vi "User_Console.vi"(8 "error in (no error)":errorcluster) -> (0 "error out":errorcluster)   [LabVIEW 2020]
doc: "Thread VIT"
uses:
  controls/Event_User.ctl
  controls/Configuration_Database.ctl
  controls/Share_Data.ctl
  <vilib>/Utility/error.llb/Error Cluster From Error Code.vi
  <vilib>/ErrorRing/Error Ring.xnode
  SubVIs/Message Queue/Message Queue.lvlib
  controls/FGV_To_Do.ctl
  Controller/User_Console_Local_Data.ctl
  Controller/User_Console_References.ctl
  SubVIs/Message Queue/Enqueue Message (Single).vi
  Controller/User_Console.ctl
panel:
  in  "User Console":T1
  # "[Covers: UI1]"
  # "[Covers: UI12A]"
  # "[Covers: UI12A1]"
  # "[Covers: UI12B]"
  # "[Covers: UI12B1]"
  # "[Covers: UI12A2]"
  # "[Covers: UI12B2]"
  # "[Covers: UI2D]"
  # "[Covers: UI2D1]"
  # "Fourth Floor"
  # "Third Floor"
  # "Second Floor"
  # "First Floor"
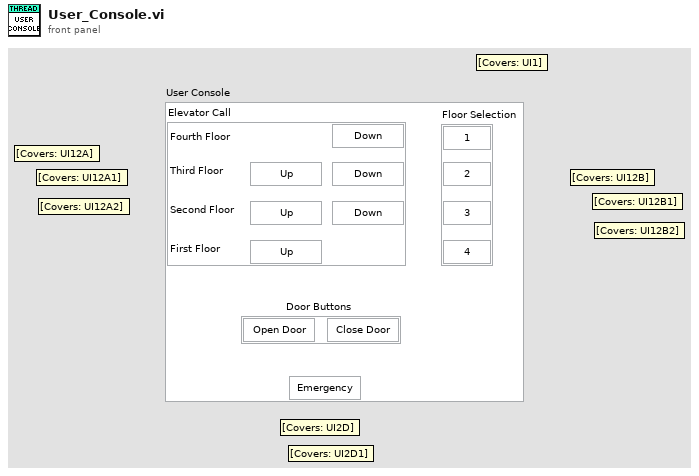
[diagram p1: front panel]
types:
  T1 = typedef "User_Console.ctl" = cluster{"Elevator Call":cluster{"Fourth Floor Down":bool, "Third Floor Down":bool, "Second Floor Down":bool, "Third Floor Up":bool, "Second Floor Up":bool, "First Floor Up":bool}, "Floor Selection":cluster{"1":bool, "2":bool, "3":bool, "4":bool}, "Door Buttons":cluster{"OpenDoor":bool, "CloseDoor":bool}, "Emergency":bool}
  T2 = typedef "FGV_To_Do.ctl" = enum16{"1 - Initialize_Events", "2 - Read_Database", "3 - Initialize QMH", "Save_Database", "Read", "4 - Close_Events", "5 - Close_QMH"}
  T3 = typedef "All_Communication_Data.ctl" = cluster{"ConfigurationDatabase":T4, "QMH":T5, "User Event":T6}
  T4 = typedef "Configuration_Database.ctl" = cluster{"DoorOpen":u8, "DoorClose":u8, "TravelTime":u8, "InactivityTime":u8}
  T5 = typedef "Message Queue.lvlib/All Message Queues.ctl" = cluster{"UserConsole":refnum<queue>, "DisplayConsole":refnum<queue>, "SensorInterface":refnum<queue>}
  T6 = typedef "Event_User.ctl" = cluster{"User Event - Stop":refnum<user-event>, "User Event - Error":refnum<user-event>}
  T7 = typedef "User_Console_Local_Data.ctl" = cluster{"Configuration_Data":T8, "UserConsole_Ref":T9, "Travel?":bool, "Terminate?":bool, "Inactivity time":dbl}
  T8 = typedef "Share_Data.ctl" = cluster{"ConfigurationDatabase":T4, "User Event":T6}
  T9 = typedef "User_Console_References.ctl" = cluster{"First Floor Up":refnum<vi>, "Second Floor Up":refnum<vi>, "Third Floor Up":refnum<vi>, "Second Floor Down":refnum<vi>, "Third Floor Down":refnum<vi>, "Fourth Floor Down":refnum<vi>, "1":refnum<vi>, "2":refnum<vi>, "3":refnum<vi>, "4":refnum<vi>, "Emergency":refnum<vi>, "CloseDoor":refnum<vi>, "OpenDoor":refnum<vi>}
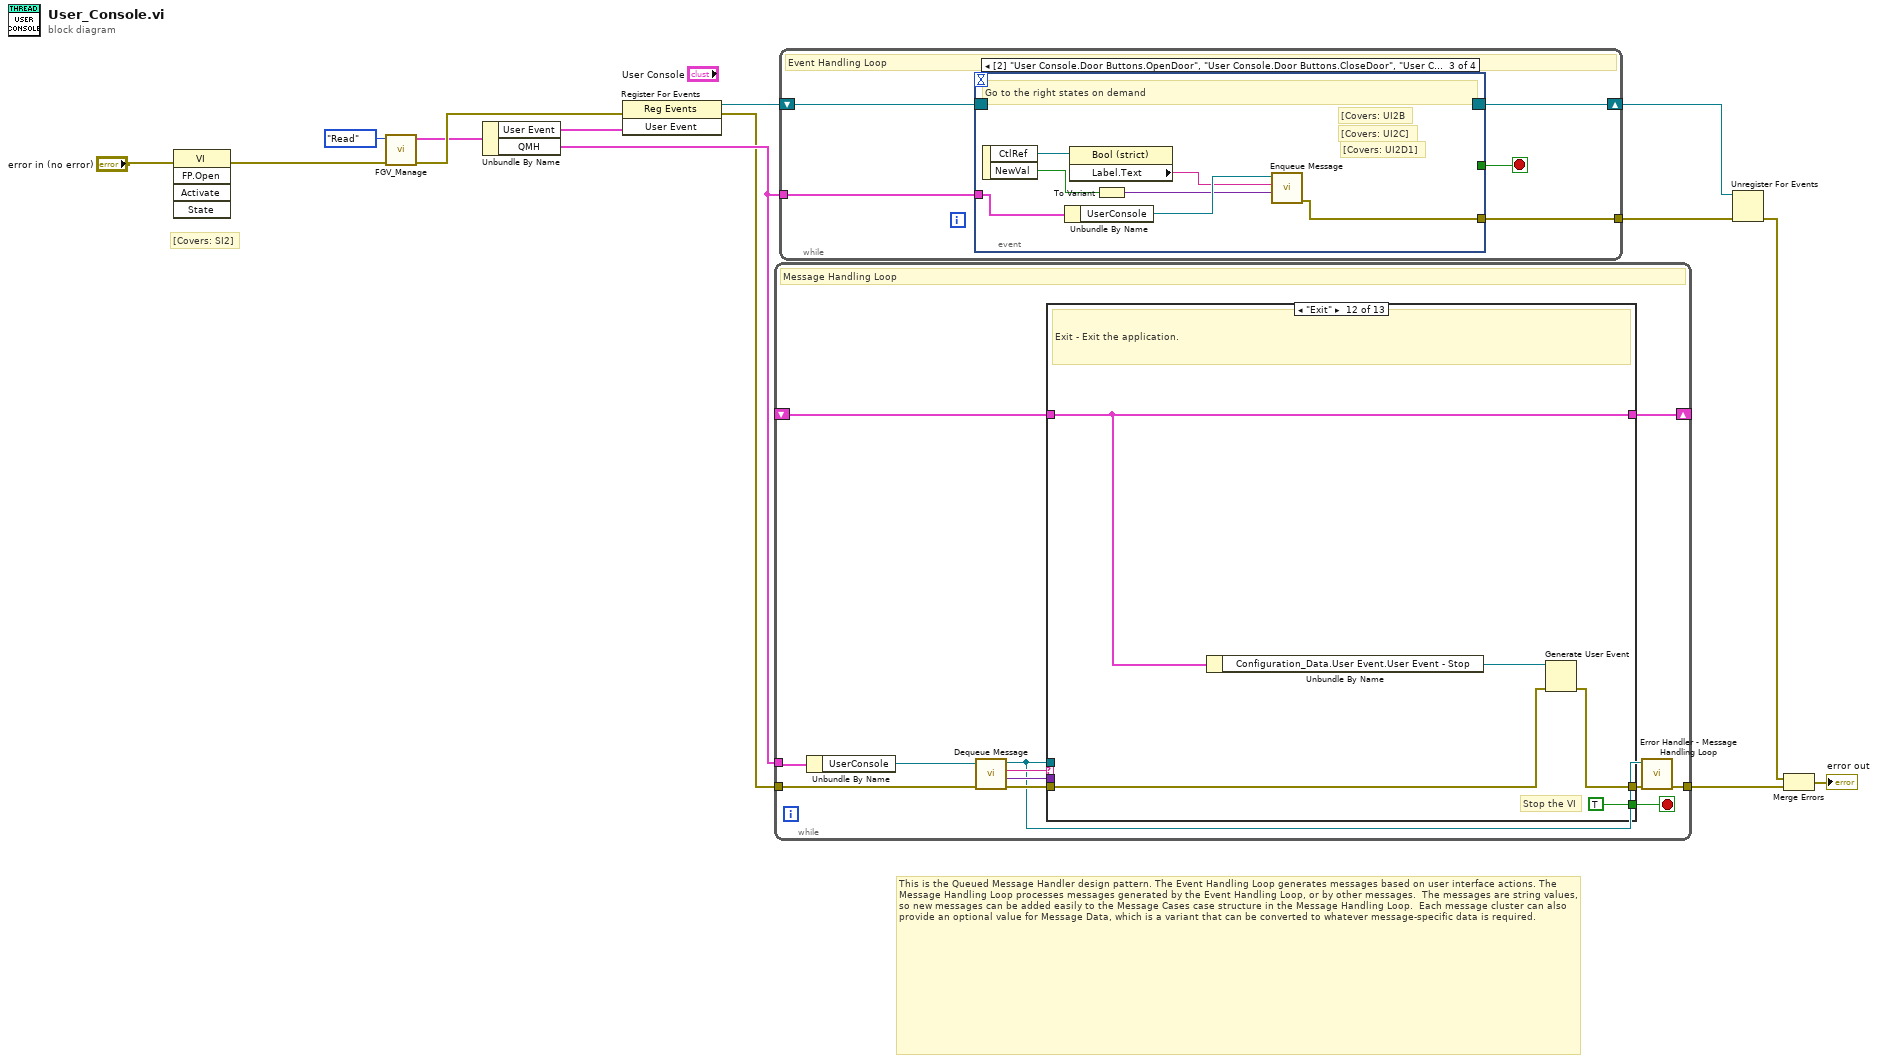
[diagram p0: block diagram]
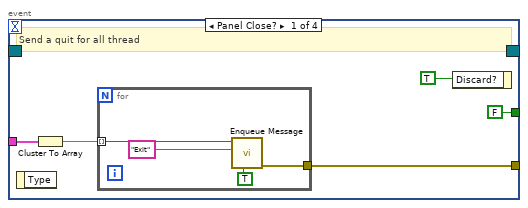
[diagram p2: hidden frame]
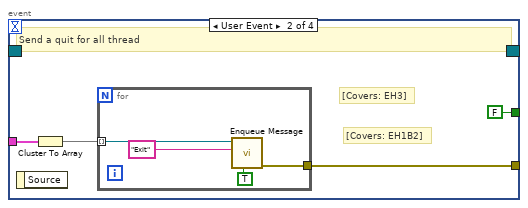
[diagram p3: hidden frame]
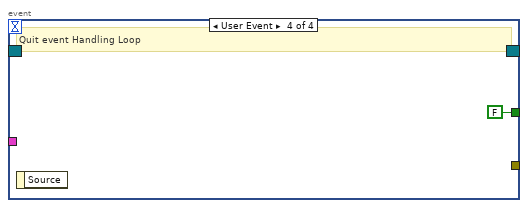
[diagram p4: hidden frame]
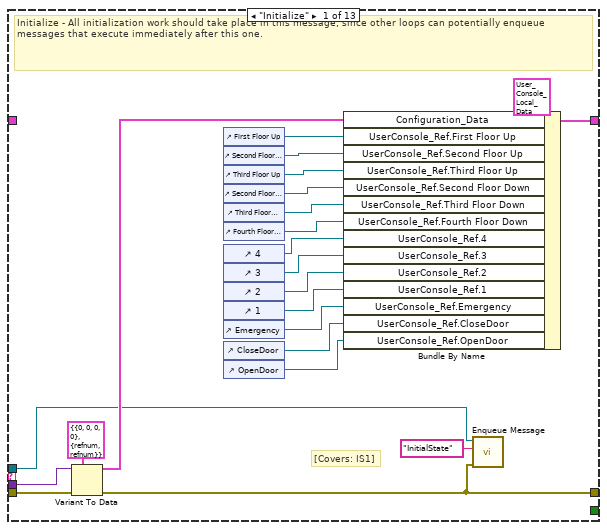
[diagram p5: hidden frame]
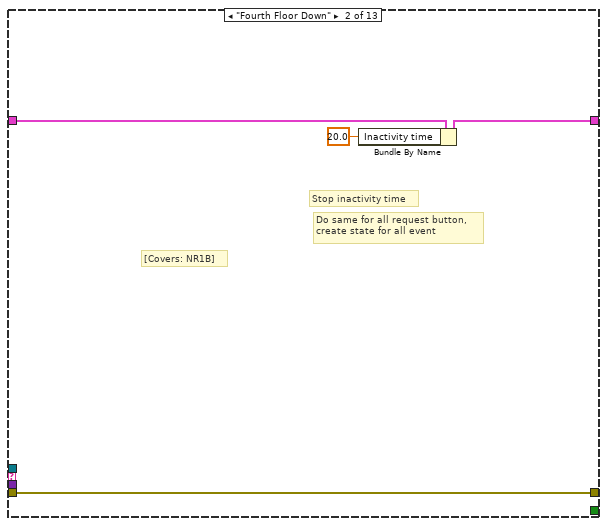
[diagram p6: hidden frame]
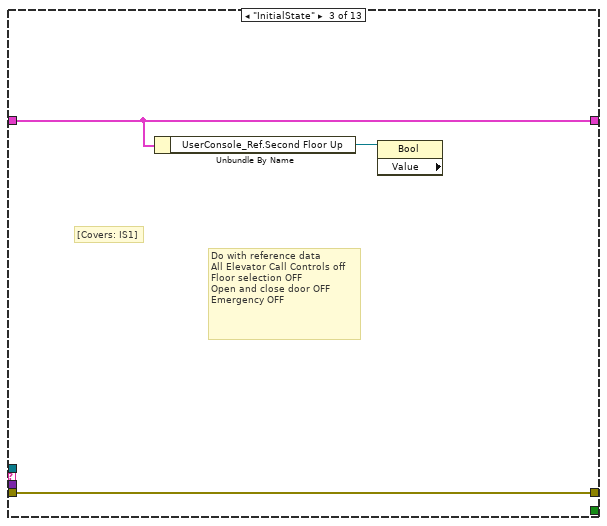
[diagram p7: hidden frame]
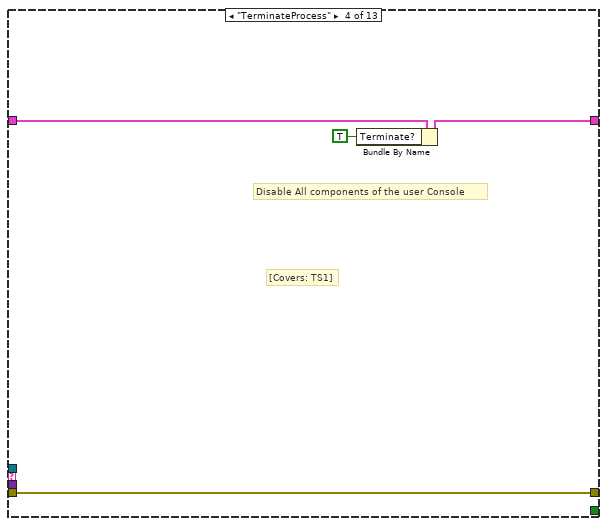
[diagram p8: hidden frame]
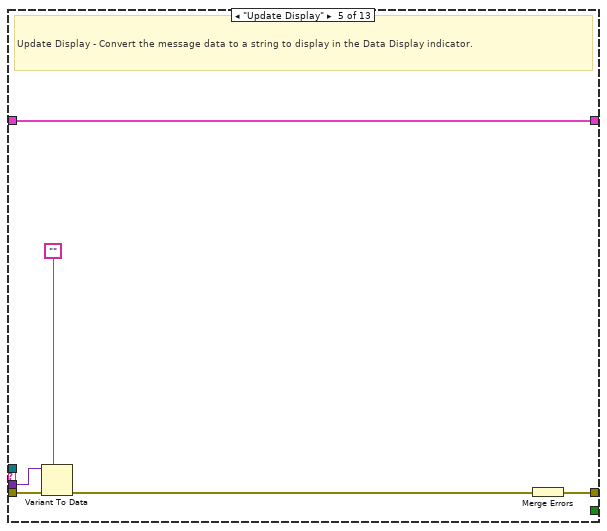
[diagram p9: hidden frame]
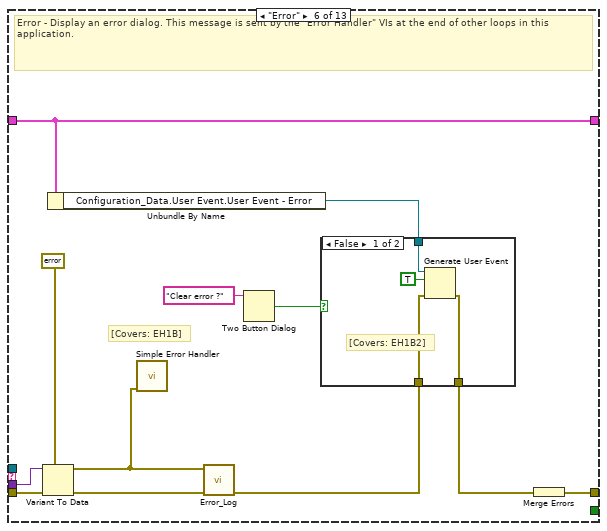
[diagram p10: hidden frame]
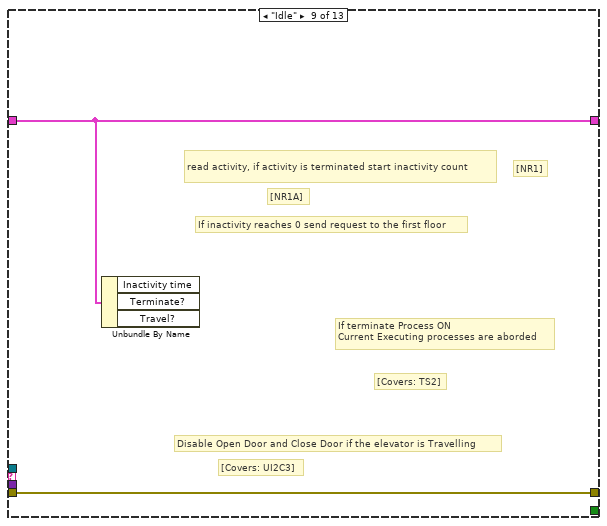
[diagram p14: hidden frame]
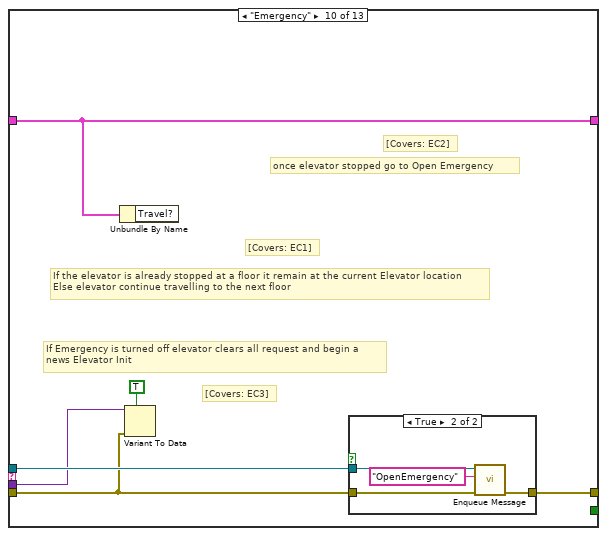
[diagram p15: hidden frame]
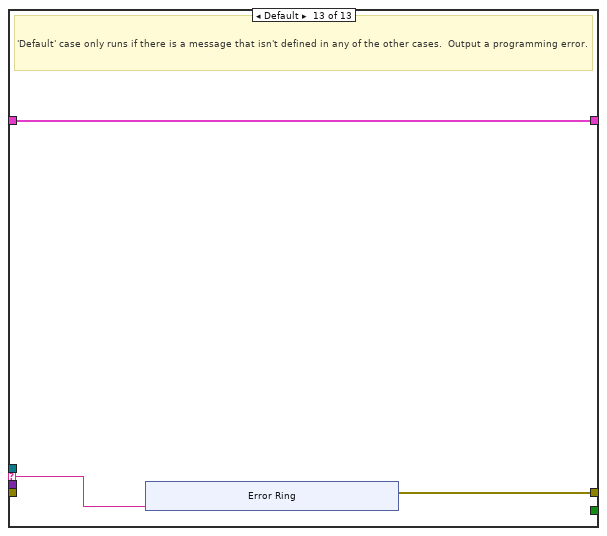
[diagram p18: hidden frame]
diagram:
  # "[Covers: SI2]"
  # "This is the Queued Message Handler design pattern. The Event Handling Loop generates messages based on user interface actions. The Message Handling Loop processes messages generated by the Event Handling Loop, or by other messages.  The messages are string values, so new messages can be added easily to the Message Cases case structure in the Message Handling Loop.  Each message cluster can also provide an optional value for Message Data, which is a variant that can be converted to whatever message-specific data is required."
  n1 = invoke class="VI" method="FP.Open"(error in="error in (no error)") -> (error out=w1:errorcluster)  [unwired: 4 in, 4 out]
  n2 = call "FGV_Manage.vi"("error in (no error)"=w1, "To do"=FGV_To_Do."Read") -> ("error out"=w11:errorcluster, "All_Communication OUT"=w9:T3)  [unwired: 8 in]
  n3 = Unbundle By Name(w9) -> ("User Event"=w10:T6, "QMH"=w13:T5)
  n4 = register-events(error in=w11, w10) -> (reference out=w7:refnum<event-registration>, error out=w12:errorcluster)  [unwired: 1 in]
  n5 = while {
    tunnel: w13 -> [w16]
    shift-right: [w25] -> _
    shift-left: _ -> [w26]
    tunnel: w12 -> [w23]
    tunnel: [w18] -> w3
    stop <- w24 stop-if-true
    # "Message Handling Loop"
    n6 = Unbundle By Name(w16) -> ("UserConsole"=w15:refnum<queue>)
    n7 = call "Dequeue Message.vi"("error in (no error)"=w23, "Message Queue"=w15) -> ("error out"=w22:errorcluster, "Message Data"=w20:variant, "Message"=w21:string, "dup Message Queue"=w19:refnum<queue>)  [unwired: 6 in]
    n8 = case "Message Cases" shown="\"Exit\"" w21 {
      selector: w21 -> [_ _ _ _ _ _ _ _ _ _ _ _ w106]
      tunnel: w19 -> [w28 _ _ _ _ _ _ _ _ w92 _ _ _]
      tunnel: w22 -> [w47 w52 w55 w59 w63 w77 w84 w86 w88 w91 w100 w102 _]
      tunnel: [w29 w52 w55 w59 w64 w74 w84 w86 w88 w93 w100 w101 w107] -> w17
      tunnel: w26 -> [_ w51 w54 w58 w65 w71 w83 w85 w87 w94 w99 w104 w108]
      tunnel: [w43 w50 w54 w57 w65 w71 w83 w85 w87 w94 w99 w104 w108] -> w25
      tunnel: [_ _ _ _ _ _ _ _ _ _ _ TRUE _] -> w24
      tunnel: w20 -> [w46 _ _ _ w62 w76 _ _ _ w90 _ _ _]
      frame "Initialize" {
        # "[Covers: IS1]"
        # "Initialize - All initialization work should take place in this message, since other loops can potentially enqueue messages that execute immediately after this one."
        n9 = Variant To Data(error in=w47, type=T8 {"ConfigurationDatabase"={"DoorOpen"=0, "DoorClose"=0, "TravelTime"=0, "InactivityTime"=0}, "User Event"={"User Event - Stop"=refnum, "User Event - Error"=refnum}} ("Share_Data"), Variant=w46) -> (data=w44:T8, error out=w29:errorcluster)
        n10 = control-ref of="First Floor Up"() -> (w42:refnum<vi>)
        n11 = control-ref of="Second Floor Up"() -> (w41:refnum<vi>)
        n12 = control-ref of="Third Floor Up"() -> (w40:refnum<vi>)
        n13 = control-ref of="Second Floor Down"() -> (w39:refnum<vi>)
        n14 = control-ref of="Third Floor Down"() -> (w38:refnum<vi>)
        n15 = control-ref of="Fourth Floor Down"() -> (w37:refnum<vi>)
        n16 = control-ref of="4"() -> (w36:refnum<vi>)
        n17 = control-ref of="3"() -> (w35:refnum<vi>)
        n18 = control-ref of="2"() -> (w34:refnum<vi>)
        n19 = control-ref of="1"() -> (w33:refnum<vi>)
        n20 = control-ref of="Emergency"() -> (w32:refnum<vi>)
        n21 = control-ref of="CloseDoor"() -> (w31:refnum<vi>)
        n22 = control-ref of="OpenDoor"() -> (w30:refnum<vi>)
        n23 = Bundle By Name(cluster=T7 {"Configuration_Data"={"ConfigurationDatabase"={"DoorOpen"=0, "DoorClose"=0, "TravelTime"=0, "InactivityTime"=0}, "User Event"={"User Event - Stop"=refnum, "User Event - Error"=refnum}}, "UserConsole_Ref"={"First Floor Up"=refnum, "Second Floor Up"=refnum, "Third Floor Up"=refnum, "Second Floor Down"=refnum, "Third Floor Down"=refnum, "Fourth Floor Down"=refnum, "1"=refnum, "2"=refnum, "3"=refnum, "4"=refnum, "Emergency"=refnum, "CloseDoor"=refnum, "OpenDoor"=refnum}, "Travel?"=FALSE, "Terminate?"=FALSE, "Inactivity time"=0.0} ("Local_Data"), "Configuration_Data"=w44, "UserConsole_Ref.First Floor Up"=w42, "UserConsole_Ref.Second Floor Up"=w41, "UserConsole_Ref.Third Floor Up"=w40, "UserConsole_Ref.Second Floor Down"=w39, "UserConsole_Ref.Third Floor Down"=w38, "UserConsole_Ref.Fourth Floor Down"=w37, "UserConsole_Ref.4"=w36, "UserConsole_Ref.3"=w35, "UserConsole_Ref.2"=w34, "UserConsole_Ref.1"=w33, "UserConsole_Ref.Emergency"=w32, "UserConsole_Ref.CloseDoor"=w31, "UserConsole_Ref.OpenDoor"=w30) -> (w43:T7)
        n24 = call-poly "Enqueue Message.vi"("error in (no error)"=w29, "Message"="InitialState", "Message Queue"=w28) -> ()  [unwired: 7 in, 2 out]
      }
      frame "Fourth Floor Down" {
        # "Do same for all request button, \ncreate state for all event"
        # "Stop inactivity time"
        # "[Covers: NR1B]"
        n25 = Bundle By Name(cluster=w51, "Inactivity time"=20.0) -> (w50:T7)
      }
      frame "InitialState" {
        # "[Covers: IS1]"
        # "Do with reference data\nAll Elevator Call Controls off\nFloor selection OFF\nOpen and close door OFF\nEmergency OFF"
        n26 = Unbundle By Name(w54) -> ("UserConsole_Ref.Second Floor Up"=w53:refnum<vi>)
        n27 = property class="Bool" props=["Value"](reference=w53) -> ()  [unwired: 1 in, 3 out]
      }
      frame "TerminateProcess" {
        # "[Covers: TS1]"
        # "Disable All components of the user Console"
        n28 = Bundle By Name(cluster=w58, "Terminate?"=TRUE) -> (w57:T7)
      }
      frame "Update Display" {
        # "Update Display - Convert the message data to a string to display in the Data Display indicator."
        n29 = Variant To Data(error in=w63, type="", Variant=w62) -> (error out=w60:errorcluster)  [unwired: 1 out]
        n30 = Merge Errors(w60) -> (w64:errorcluster)
      }
      frame "Error" {
        # "[Covers: EH1B]"
        # "Error - Display an error dialog. This message is sent by the \"Error Handler\" VIs at the end of other loops in this application."
        n31 = Variant To Data(error in=w77, type=errorcluster {"status"=FALSE, "code"=0, "source"=""} ("error constant"), Variant=w76) -> (data=w72:errorcluster, error out=w73:errorcluster)
        n32 = Unbundle By Name(w71) -> ("Configuration_Data.User Event.User Event - Error"=w70:refnum<user-event>)
        n33 = call <vilib>:"Simple Error Handler.vi"("error in (no error)"=w72) -> ()  [unwired: 4 in, 5 out]
        n34 = call "Error_Log.vi"("error in"=w73, "Error report"=w72) -> ("error out"=w67:errorcluster)  [unwired: 9 in]
        n35 = Two Button Dialog(message="Clear error ?") -> (T button?=w69:bool)  [unwired: 2 in]
        n36 = case shown="False" w69 {
          tunnel: w70 -> [w81 _]
          tunnel: w67 -> [w79 w82]
          tunnel: [w78 w82] -> w66
          frame False {
            # "[Covers: EH1B2]"
            n37 = Generate User Event(user event=w81, event data cluster=TRUE ("event data"), error in=w79) -> (error out=w78:errorcluster)  [unwired: 1 in, 1 out]
          }
          frame True {
            # "[Covers: EH1B1]"
          }
        }
        n38 = Merge Errors(w66) -> (w74:errorcluster)
      }
      frame "OpenDoor" {
        # "[Covers: UI2C1]"
        # "Open Door when the elevator is stopped on a floor"
      }
      frame "CloseDoor" {
        # "[Covers: UI2C2]"
        # "Close Door when the elevator is stopped on a floor"
      }
      frame "Idle" {
        # "read activity, if activity is terminated start inactivity count"
        # "[NR1A]"
        # "If inactivity reaches 0 send request to the first floor"
        # "[NR1]"
        # "[Covers: TS2]"
        # "If terminate Process ON\nCurrent Executing processes are aborded"
        # "Disable Open Door and Close Door if the elevator is Travelling"
        # "[Covers: UI2C3]"
        n39 = Unbundle By Name(w87) -> ()  [unwired: 3 out]
      }
      frame "Emergency" {
        # "[Covers: EC3]"
        # "If Emergency is turned off elevator clears all request and begin a \nnews Elevator Init"
        # "once elevator stopped go to Open Emergency"
        # "[Covers: EC2]"
        # "If the elevator is already stopped at a floor it remain at the current Elevator location\nElse elevator continue travelling to the next floor"
        # "[Covers: EC1]"
        n40 = Unbundle By Name(w94) -> ()  [unwired: 1 out]
        n41 = Variant To Data(error in=w91, type=TRUE, Variant=w90) -> ()  [unwired: 2 out]
        n42 = case shown="True" {
          selector: _ -> [_ _]
          tunnel: [_ w98] -> w93
          tunnel: w92 -> [_ w97]
          tunnel: w91 -> [_ w95]
          frame False {
          }
          frame True {
            n43 = call-poly "Enqueue Message.vi"("error in (no error)"=w95, "Message"="OpenEmergency", "Message Queue"=w97) -> ("error out"=w98:errorcluster)  [unwired: 7 in, 1 out]
          }
        }
      }
      frame "OpenEmergency" {
        # "Door Open and remain Open"
        # "[Covers: EC2]"
      }
      frame "Exit" {
        # "Stop the VI"
        # "Exit - Exit the application."
        n44 = Unbundle By Name(w104) -> ("Configuration_Data.User Event.User Event - Stop"=w103:refnum<user-event>)
        n45 = Generate User Event(user event=w103, error in=w102) -> (error out=w101:errorcluster)  [unwired: 2 in, 1 out]
      }
      frame Default {
        # "'Default' case only runs if there is a message that isn't defined in any of the other cases.  Output a programming error."
        n46 = xnode "Error Ring"("parameter 0"=w106) -> ("error out"=w107:errorcluster)
      }
    }
    n47 = call "Error Handler - Message Handling Loop.vi"("error in (no error)"=w17, "Message Queue"=w19) -> ("dup error in"=w18:errorcluster)  [unwired: 8 in, 1 out]
  }
  n48 = while {
    tunnel: w13 -> [w120]
    shift-right: [w118] -> w5
    shift-left: w7 -> [w119]
    tunnel: [w116] -> w6
    stop <- w117 stop-if-true
    # "Event Handling Loop"
    n49 = event shown="[2] \"User Console.Door Buttons.OpenDoor\", \"User Console.Door Buttons.CloseDoor\", \"User Console.Emergency\", \"User Console.Floor Selection.1\", \"User Console.Floor Selection.2\", \"User Console.Floor Selection.3\", \"User Console.Floor Selection.4\": Value Change" {
      selector: w119 -> [_ _ _ _]
      dyn-events: [_ _ _ _] -> w118
      timeout: _ -> [_ _ _ _]
      tunnel: [FALSE ("Discard?") FALSE ("Discard?") _ FALSE ("Discard?")] -> w117
      tunnel: w120 -> [w124 w133 w143 _]
      tunnel: [w123 w132 w140 _] -> w116
      event Panel Close? {
        # "Send a quit for all thread"
        n50 = event-data() -> ()  [unwired: 1 in, 1 out]
        n51 = Cluster To Array(cluster=w124) -> (array=w122:refnum<queue>[])
        n52 = for {
          tunnel: w122 -> [w129] mode=indexing
          tunnel: [w128] -> w123
          n53 = call-poly "Enqueue Message.vi"("Priority Message? (F)"=TRUE, "Message"="Exit", "Message Queue"=w129) -> ("error out"=w128:errorcluster)  [unwired: 7 in, 1 out]
        }
        n54 = event-data("Discard?"=TRUE) -> ()  [unwired: 1 in, 1 out]
      }
      event User Event {
        # "[Covers: EH3]"
        # "[Covers: EH1B2]"
        # "Send a quit for all thread"
        n55 = event-data() -> ()  [unwired: 1 in, 1 out]
        n56 = Cluster To Array(cluster=w133) -> (array=w131:refnum<queue>[])
        n57 = for {
          tunnel: w131 -> [w137] mode=indexing
          tunnel: [w136] -> w132
          n58 = call-poly "Enqueue Message.vi"("Priority Message? (F)"=TRUE, "Message"="Exit", "Message Queue"=w137) -> ("error out"=w136:errorcluster)  [unwired: 7 in, 1 out]
        }
      }
      event Value Change {
        # "[Covers: UI2B"
        # "[Covers: UI2C]"
        # "[Covers: UI2D1]"
        # "Go to the right states on demand"
        n59 = event-data() -> ("CtlRef"=w144:refnum<vi>, "NewVal"=w139:bool)  [unwired: 1 in]
        n60 = Unbundle By Name(w143) -> ("UserConsole"=w142:refnum<queue>)
        n61 = property class="Bool (strict)"(reference=w144) -> ("Label.Text"=w141:string)  [unwired: 1 in, 2 out]
        n62 = To Variant(anything=w139) -> (Variant=w138:variant)
        n63 = call-poly "Enqueue Message.vi"("Message Data"=w138, "Message"=w141, "Message Queue"=w142) -> ("error out"=w140:errorcluster)  [unwired: 7 in, 1 out]
      }
      event User Event {
        # "Quit event Handling Loop"
        n64 = event-data() -> ()  [unwired: 1 in, 1 out]
      }
    }
  }
  n65 = Unregister For Events(event registration refnum=w5, error in=w6) -> (error out=w4:errorcluster)
  n66 = Merge Errors(w4, w3) -> (→"error out":errorcluster)
